vi "Create.vi"() -> (7 "Historian Identity out":refnum<class "Historian Identity.lvclass">)   [LabVIEW 2020, in "VolatusHistorian.lvlib" / "Historian Identity.lvclass"]
uses:
  Historian Identity.lvclass
  Historian Identity.lvclass/Historian Identity.ctl
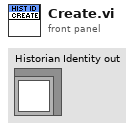
[diagram p1: front panel]
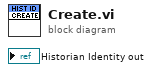
[diagram p0: block diagram]
diagram:
